vi "Test Execute SQL Query (blob as string).vi"(8 "error in (no error)":errorcluster, 10 "query":string, 11 "database in":path) -> (0 "error out":errorcluster, 1 "Query Result":string[][](array[string]), 2 "nonzero result?":bool=TRUE)   [LabVIEW 2020, in "sqlite3.lvlib"]
uses:
  sqlite3.lvlib
  sqlite/VIs/open v2.vi
  sqlite/VIs/prepare v2.vi
  sqlite/VIs/step.vi
  sqlite/VIs/column count.vi
  compound/Column.vi
  compound/Resolve Result Type.vi
  sqlite/VIs/finalize.vi
  sqlite/VIs/close v2.vi
  sqlite/subvi/Error Converter (ErrCode or Status).vi
  sqlite/VIs/column text.vi
  sqlite/VIs/column bytes.vi
  sqlite/VIs/column blob.vi
  utilities/MoveBlock.vi
  sqlite/VIs/column type.vi
  sqlite/VIs/errstr.vi
panel:
  out "Pictures":picture[](array[picture])
  in  "desired return type":string
  # "can only read columns as blobs if they are created \nas blobs.  trying to read another column affinity as a blob won't work"
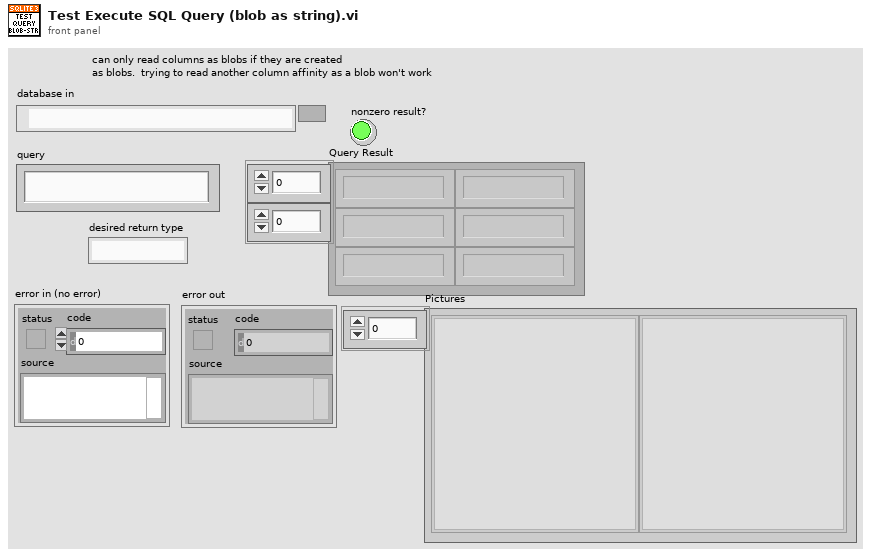
[diagram p1: front panel]
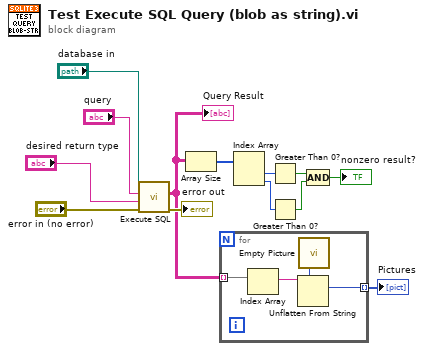
[diagram p0: block diagram]
diagram:
  n1 = call "Execute SQL.vi"("error in (no error)"="error in (no error)", "[disabled] return type (string)"="desired return type", "sql (string)"="query", "database in"="database in") -> ("error out"=→"error out":errorcluster, "Query Result"=w6:string[][])  [unwired: 6 in]
  "Query Result" <- w6
  n2 = Array Size(array=w6) -> (size(s)=w12:i32[])
  n3 = for {
    tunnel: w6 -> [w17] mode=indexing
    tunnel: [w14] -> w5 mode=indexing
    n4 = Index Array(array=w17) -> (element=w16:string)  [unwired: 1 in]
    n5 = call "Empty Picture"() -> ("empty picture"=w15:picture)
    n6 = Unflatten From String(type=w15, binary string=w16) -> (value=w14:picture)  [unwired: 3 in, 2 out]
  }
  "Pictures" <- w5
  n7 = Index Array(array=w12) -> (element #1=w11:i32, element #2=w10:i32)  [unwired: 2 in]
  n8 = Greater Than 0?(x=w11) -> (x > 0?=w9:bool)
  n9 = Greater Than 0?(x=w10) -> (x > 0?=w8:bool)
  n10 = Compound Arithmetic op=AND(w9, w8) -> (→"nonzero result?":bool)
